vi "Setup.vi"(8 "error in (no error)":errorcluster, 11 "UnitTestFramework in":refnum<class "UnitTestFramework.lvclass">) -> (0 "error out":errorcluster, 3 "UnitTestFramework out":refnum<class "UnitTestFramework.lvclass">)   [LabVIEW 2019, in "UnitTestFramework.lvclass"]
uses:
  UnitTestFramework.lvclass
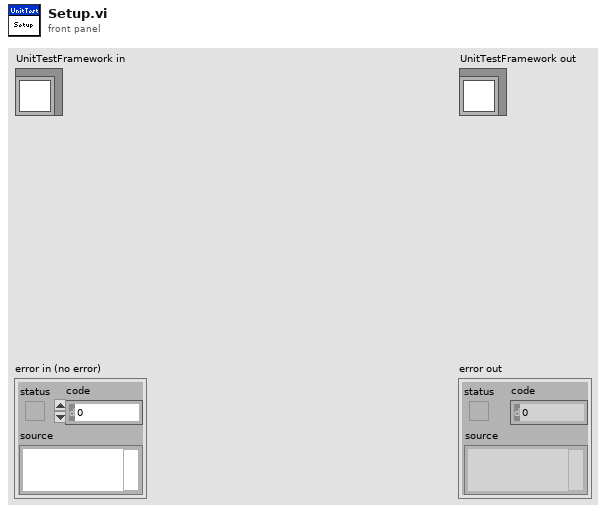
[diagram p1: front panel]
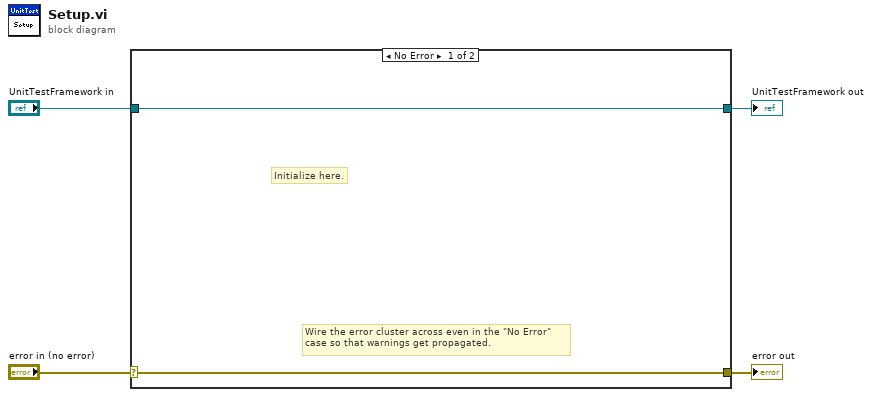
[diagram p0: block diagram]
diagram:
  n1 = case shown="No Error" "error in (no error)" {
    selector: "error in (no error)" -> [w5 w8]
    tunnel: [w5 w8] -> w3
    tunnel: [w6 w7] -> w1
    tunnel: "UnitTestFramework in" -> [w6 w7]
    frame No Error {
      # "Initialize here."
      # "Wire the error cluster across even in the \"No Error\"\ncase so that warnings get propagated."
    }
    frame Error {
    }
  }
  "error out" <- w3
  "UnitTestFramework out" <- w1
